vi "Compile Auto Path.vi"(9 "Scale Right?":bool, 10 "Switch Right?":bool, 11 "Start Left?":bool) -> (3 "Auto Paths":path[](array[path]))   [LabVIEW 2017]
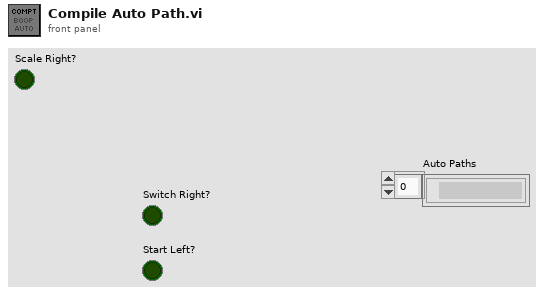
[diagram p1: front panel]
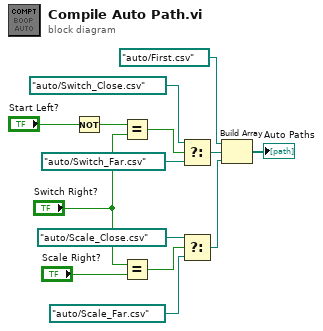
[diagram p0: block diagram]
diagram:
  n1 = Not(x="Start Left?") -> (.not. x?=w13:bool)
  n2 = Equal?(x=w13, y="Switch Right?") -> (x = y?=w12:bool)
  n3 = Equal?(x="Switch Right?", y="Scale Right?") -> (x = y?=w7:bool)
  n4 = Select(t=path "/auto/Switch_Close.csv", s=w12, f=path "/auto/Switch_Far.csv") -> (s? t:f=w2:path)
  n5 = Select(t=path "/auto/Scale_Close.csv", s=w7, f=path "/auto/Scale_Far.csv") -> (s? t:f=w1:path)
  n6 = Build Array(path "/auto/First.csv", w2, w1) -> (→"Auto Paths":path[])
